vi "ProcessQuerry.vi"(7 "Isa Module ID":i32=-1, 8 "error in (no error)":errorcluster, 9 "Module ID":i32, 10 "Data Cluster in":T1, 11 "Delacor_lib_QMH_Message Queue in":refnum<class "Delacor_lib_QMH_Message Queue.lvclass">) -> (0 "error out":errorcluster, 2 "Data Cluster 3":T1, 3 "Command":string)   [LabVIEW 2015, in "ISA010_module.lvlib"]
uses:
  ISA010_module.lvlib
  <vilib>/Delacor/Delacor QMH/Libraries/Message Queue_class/Delacor_lib_QMH_Message Queue.lvclass
  Module Data--cluster.ctl
  ISA010/ISA010.lvclass
  libraries/ModBUS.lvlibp/Base/Modbus.lvclass
  ISA010/Command.ctl
  <vilib>/Delacor/Delacor QMH/Libraries/Message Queue_class/Delacor_lib_QMH_Enqueue Message (Single).vi
  libraries/Serializer.lvlibp
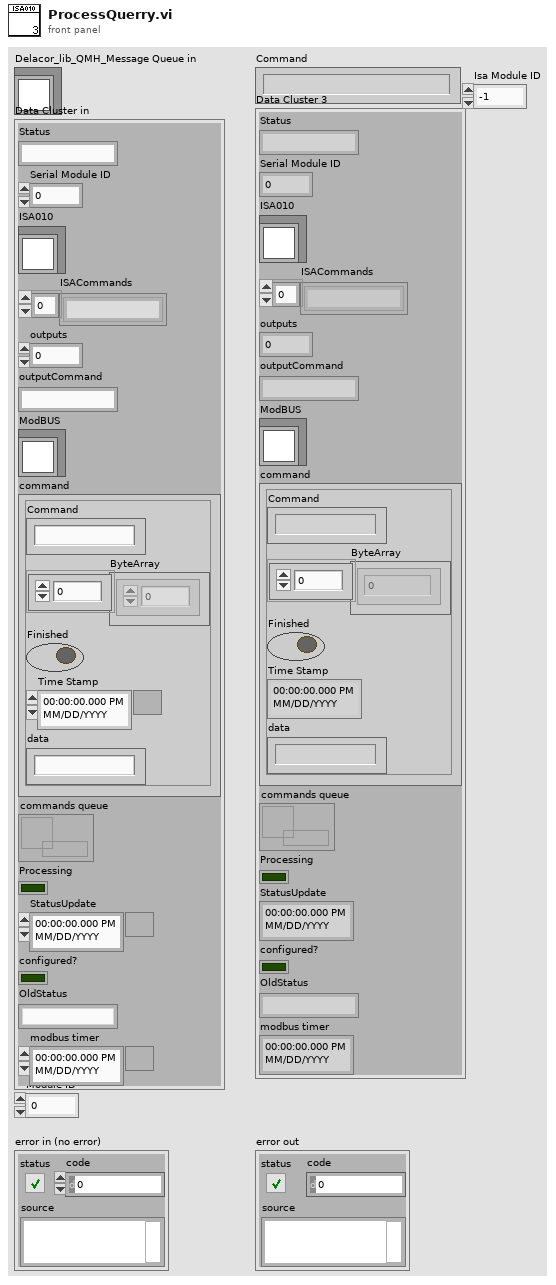
[diagram p1: front panel]
types:
  T1 = typedef "ISA010_module.lvlib/Module Data--cluster.ctl" = cluster{"Status":string, "Serial Module ID":i32, "ISA010":refnum<class "ISA010.lvclass">, "ISACommands":string[], "outputs":u16, "outputCommand":string, "ModBUS":refnum<class "Modbus.lvclass">, "command":T2, "commands queue":refnum<queue>, "Processing":bool, "StatusUpdate":timestamp, "configured?":bool, "OldStatus":string, "modbus timer":timestamp}
  T2 = typedef "Command.ctl" = cluster{"Command":string, "ByteArray":u8[], "Finished":bool, "Time Stamp":timestamp, "data":string}
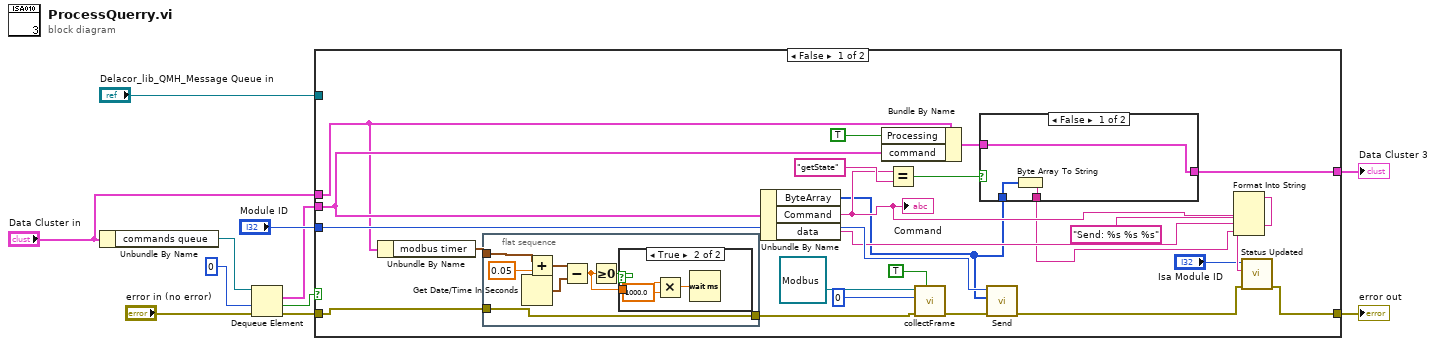
[diagram p0: block diagram]
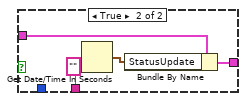
[diagram p3: hidden frame]
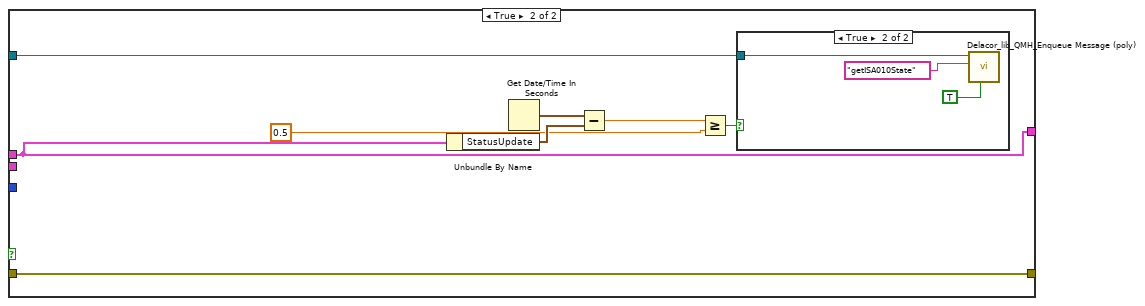
[diagram p4: hidden frame]
diagram:
  n1 = Unbundle By Name("Data Cluster in") -> ("commands queue"=w11:refnum<queue>)
  n2 = Dequeue Element(queue=w11, timeout in ms (-1)=0, error in (no error)="error in (no error)") -> (element=w8:T2, timed out?=w5:bool, error out=w6:errorcluster)  [unwired: 1 out]
  n3 = case shown="False" w5 {
    tunnel: [w30 w54] -> w2
    tunnel: "Data Cluster in" -> [w15 w54]
    tunnel: [w21 w60] -> w4
    tunnel: w6 -> [w14 w60]
    tunnel: w8 -> [w34 _]
    tunnel: "Module ID" -> [w29 _]
    tunnel: "Delacor_lib_QMH_Message Queue in" -> [_ w53]
    frame False {
      n4 = Unbundle By Name(w15) -> ("modbus timer"=w13:timestamp)
      n5 = flat-sequence {
        tunnel: w14 -> [w38]
        tunnel: w13 -> [w42]
        tunnel: [w38] -> w12
        frame #0 {
          n6 = Get Date/Time In Seconds() -> (seconds since 1Jan1904=w36:timestamp)
          n7 = Add(x=w42, y=0.05) -> (x+y=w37:timestamp)
          n8 = Subtract(x=w37, y=w36) -> (x-y=w39:dbl)
          n9 = Greater Or Equal To 0?(x=w39) -> (x >= 0?=w40:bool)
          n10 = case shown="True" w40 {
            tunnel: w39 -> [_ w45]
            frame False {
            }
            frame True {
              n11 = Multiply(x=w45, y=1000.0) -> (x*y=w43:dbl)
              n12 = Wait (ms)(milliseconds to wait=w43) -> ()  [unwired: 1 out]
            }
          }
        }
      }
      n13 = Unbundle By Name(w34) -> ("ByteArray"=w17:u8[], "Command"=w20:string, "data"=w19:string)
      "Command" <- w20
      n14 = Bundle By Name(cluster=w15, "Processing"=TRUE, "command"=w34) -> (w31:T1)
      n15 = Equal?(x=w20, y="getState") -> (x = y?=w32:bool)
      n16 = call-dynamic "collectFrame.vi"("Reset"=TRUE, "error in (no error)"=w12, "byte"=u8 0, "Modbus in"=refnum<class "Modbus.lvclass"> refnum) -> ("error out"=w26:errorcluster)  [unwired: 3 in, 4 out]
      n17 = case shown="False" w32 {
        tunnel: w31 -> [w48 w52]
        tunnel: [w48 w51] -> w30
        tunnel: w17 -> [w47 _]
        tunnel: [w46 "" ("string")] -> w16
        frame False {
          n18 = Byte Array To String(unsigned byte array=w47) -> (string=w46:string)
        }
        frame True {
          n19 = Get Date/Time In Seconds() -> (seconds since 1Jan1904=w50:timestamp)
          n20 = Bundle By Name(cluster=w52, "StatusUpdate"=w50) -> (w51:T1)
        }
      }
      n21 = call "Send.vi"("error in (no error)"=w26, "Bytes"=w17, "Module ID"=w29) -> ("error out"=w22:errorcluster)  [unwired: 8 in]
      n22 = Format Into String(format string="Send: %s %s %s", w20, w19, w16) -> (resulting string=w23:string)  [unwired: 2 in, 1 out]
      n23 = call "Status Updated.vi"("error in (no error)"=w22, "Status"=w23, "Module ID"="Isa Module ID") -> ("error out"=w21:errorcluster)  [unwired: 8 in]
    }
    frame True {
      n24 = Unbundle By Name(w54) -> ("StatusUpdate"=w58:timestamp)
      n25 = Get Date/Time In Seconds() -> (seconds since 1Jan1904=w59:timestamp)
      n26 = Subtract(x=w59, y=w58) -> (x-y=w57:dbl)
      n27 = Greater Or Equal?(x=w57, y=0.5) -> (x >= y?=w55:bool)
      n28 = case shown="True" w55 {
        tunnel: w53 -> [_ w63]
        frame False {
        }
        frame True {
          n29 = call-poly <vilib>:"Delacor_lib_QMH_Enqueue Message (poly).vi"("Priority Message? (F)"=TRUE, "Message"="getISA010State", "Message Queue in"=w63) -> ()  [unwired: 7 in, 2 out]
        }
      }
    }
  }
  "error out" <- w4
  "Data Cluster 3" <- w2
